vi "valid dotted ip.vi"(11 "IP Address":string) -> (3 "dotted ip":bool)   [LabVIEW 2020]
uses:
  <vilib>/regexp/Match Regular Expression.xnode
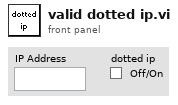
[diagram p1: front panel]
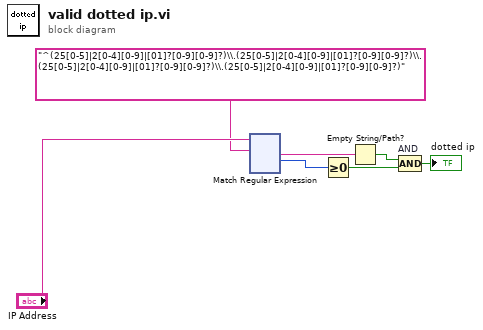
[diagram p0: block diagram]
diagram:
  n1 = xnode "Match Regular Expression"("input string"="IP Address", "regular expression"="^(25[0-5]|2[0-4][0-9]|[01]?[0-9][0-9]?)\\.(25[0-5]|2[0-4][0-9]|[01]?[0-9][0-9]?)\\.(25[0-5]|2[0-4][0-9]|[01]?[0-9][0-9]?)\\.(25[0-5]|2[0-4][0-9]|[01]?[0-9][0-9]?)") -> ("after match"=w4:string, "offset past match"=w2:i32)  [unwired: 4 in, 3 out]
  n2 = Greater Or Equal To 0?(x=w2) -> (x >= 0?=w3:bool)
  n3 = Empty String/Path?(string/path=w4) -> (empty?=w5:bool)
  n4 = Compound Arithmetic op=AND "AND"(w5, w3) -> (→"dotted ip":bool)
